vi "Reg Events of Boolean.vi"(11 "VI in":refnum<vi>) -> (3 "Event Registration Refnum out":refnum<event-registration>)   [LabVIEW 2020, in "Popup Dialog.lvlib"]
uses:
  Popup Dialog.lvlib
panel:
  out "Array":string[](array[string])
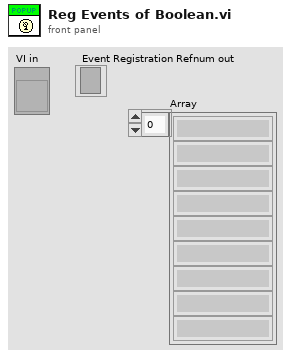
[diagram p1: front panel]
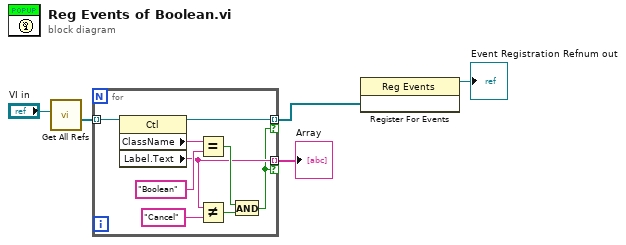
[diagram p0: block diagram]
diagram:
  n1 = call "Get All Refs.vi"("This VI"="VI in") -> ("Controls[]"=w1:refnum<vi>[])  [unwired: 8 in, 2 out]
  n2 = for {
    tunnel: w1 -> [w14] mode=indexing
    tunnel: [w13] -> w4 mode=indexing if=w6
    tunnel: [w8] -> w3 mode=indexing if=w6
    n3 = property class="Ctl"(reference=w14) -> (reference out=w13:refnum<vi>, "ClassName"=w7:string, "Label.Text"=w8:string)  [unwired: 1 in, 1 out]
    n4 = Equal?(x=w7, y="Boolean") -> (x = y?=w11:bool)
    n5 = Not Equal?(x=w8, y="Cancel") -> (x != y?=w9:bool)
    n6 = And(x=w11, y=w9) -> (x .and. y?=w6:bool)
  }
  "Array" <- w3
  n7 = register-events(w4) -> (reference out=→"Event Registration Refnum out":refnum<event-registration>)  [unwired: 2 in, 1 out]
